vi "mod_Continuous BB-QAM generation.vi"(0 "Bit stream":T1(tab), 1 "Symbol Rate, Hz":dbl=1.0 format="%.2f", 2 "QAM system parameters":T2={"samples per symbol (16)"=16, "symbol map"=[]} {"symbol map" format="%.3f"}, 5 "PN Sequence Order":i32=9, 9 "user base bit pattern":i8[](array[numeric]), 11 "error in (no error)":errorcluster, 12 "filter parameters":T3={"Alpha"=0.5, "Filter Length"=6, "TX Filter"=enum."Root Raised Cos"} {"Alpha" format="%.2f"}, 13 "Path":path) -> (4 "output complex waveform":T4 {"Y" format="%.3f"; "dt" format="%^.2e"; "t0" format="%.4f"}, 6 "modulated bitstream":i8[](array[numeric]), 8 "pulse shaping filter coefficients":dbl[](array[numeric]) format="%.2f", 10 "matched filter coefficients":dbl[](array[numeric]) format="%.2f", 15 "error out":errorcluster)   [LabVIEW 2020, in "niDMT.lvlib"]
uses:
  <vilib>/addons/Modulation/niDMT.lvlib
  <vilib>/addons/Modulation/Analog/controls/Complex Data Waveform.ctl
  <vilib>/addons/Modulation/Digital/Support/Controls/QAM System Parameters.ctl
  <vilib>/addons/Modulation/Digital/General/MT Generate Bits (Galois, PN Order).vi
  <vilib>/addons/Modulation/Digital/Support/Common/Validators/mod_Generate Bits Validate.vi
  <vilib>/addons/Modulation/Analog/support/mod_Set Error Source.vi
  <vilib>/addons/Modulation/Digital/General/subVIs/mod_Generate Bits PN Sequence.vi
  <vilib>/addons/Modulation/Digital/General/MT Generate Bits (User Defined).vi
  <vilib>/Utility/file.llb/Read From Spreadsheet File (DBL).vi
  <vilib>/addons/Modulation/Digital/Support/Common/Validators/mod_Generate Filter Coefficients Validate.vi
  <vilib>/addons/Modulation/Digital/General/subVIs/mod_Generate Filter Coefficients.vi
  <vilib>/addons/Modulation/niAMT.lvlib
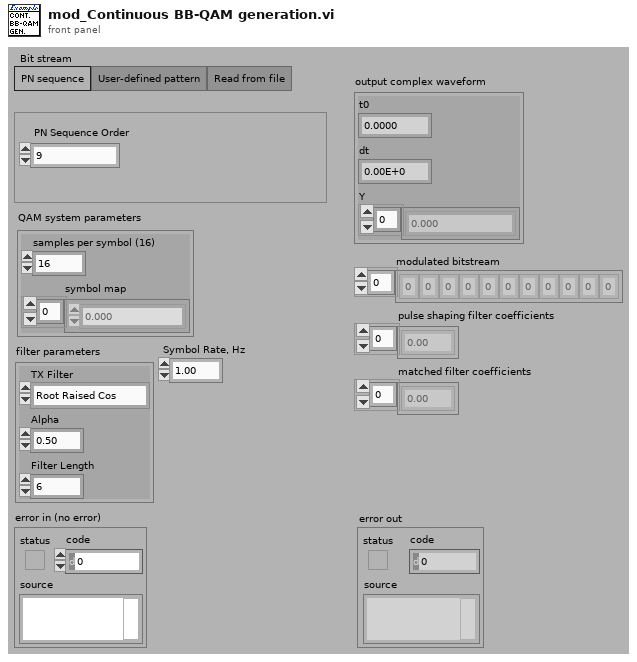
[diagram p1: front panel]
types:
  T1 = enum32{"PN sequence", "User-defined pattern", "Read from file"}
  T2 = typedef "niDMT.lvlib/QAM System Parameters.ctl" = cluster{"samples per symbol (16)":i32, "symbol map":cdb[]}
  T3 = cluster{"Alpha":dbl, "Filter Length":i32, "TX Filter":enum16{"none", "Raised Cosine", "Root Raised Cos", "Gaussian"}}
  T4 = typedef "niAMT.lvlib/Complex Data Waveform.ctl" = cluster{"t0":dbl, "dt":dbl, "Y":cdb[]}
  T5 = enum16{"none", "Raised Cosine", "Root Raised Cos", "Gaussian"}
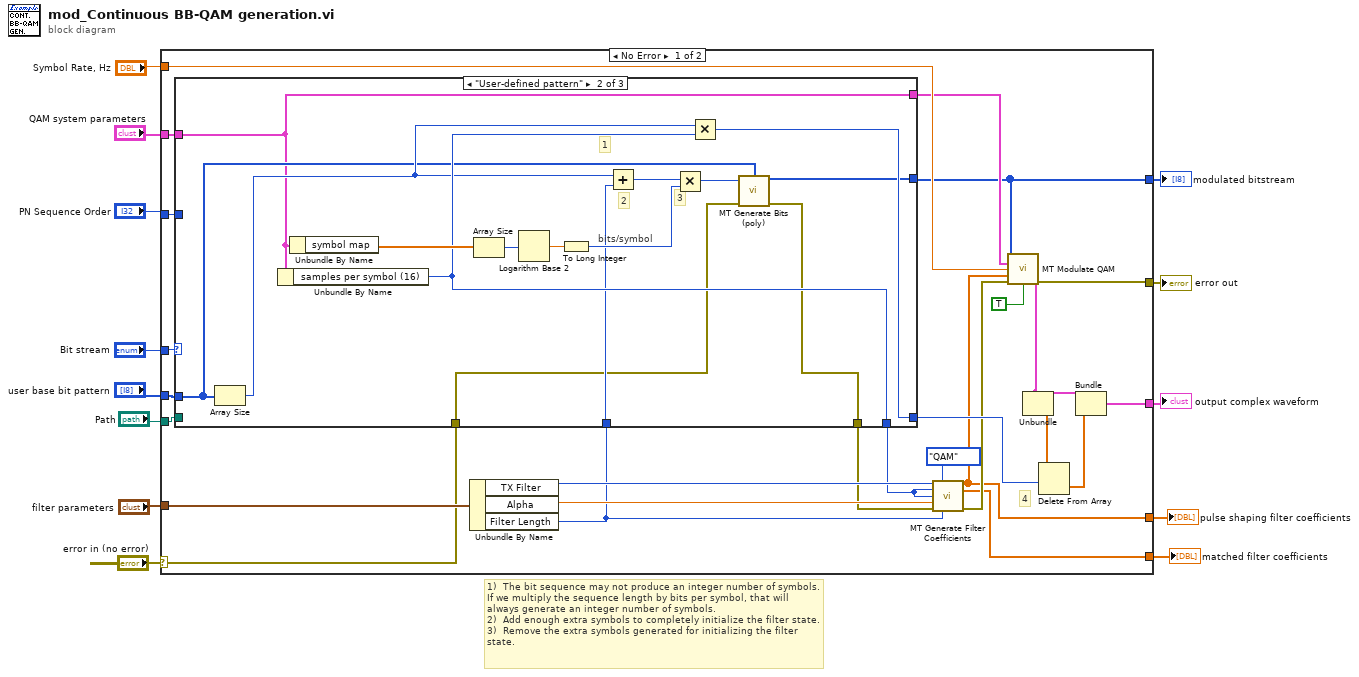
[diagram p0: block diagram]
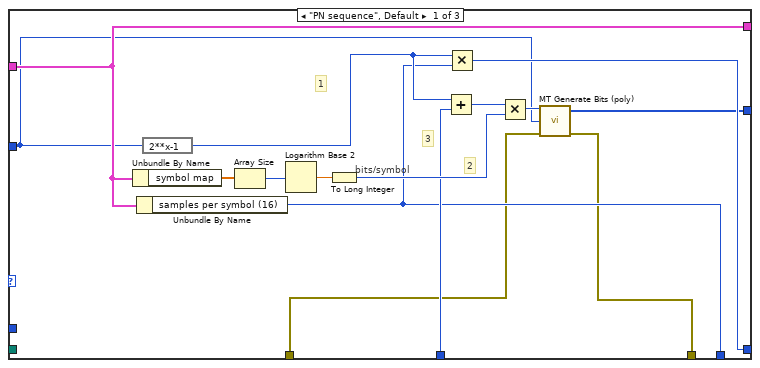
[diagram p2: hidden frame]
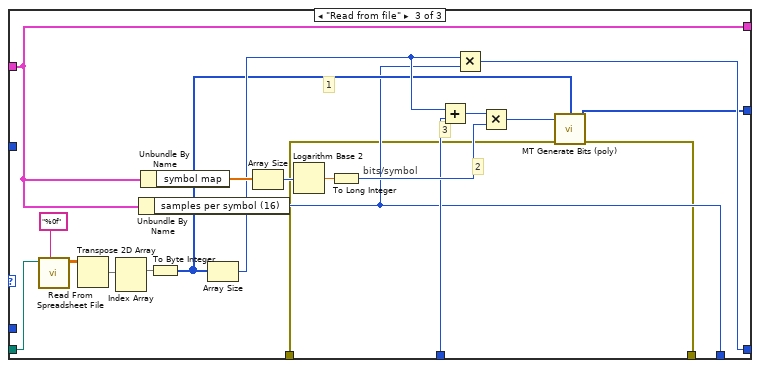
[diagram p3: hidden frame]
diagram:
  # "1)  The bit sequence may not produce an integer number of symbols.  If we multiply the sequence length by bits per symbol, that will always generate an integer number of symbols. \n2)  Add enough extra symbols to completely initialize the filter state.\n3)  Remove the extra symbols generated for initializing the filter state."
  n1 = case shown="No Error" "error in (no error)" {
    selector: "error in (no error)" -> [w19 w90]
    tunnel: [w39 _] -> w13
    tunnel: [w38 w90] -> w12
    tunnel: "Symbol Rate, Hz" -> [w35 _]
    tunnel: "PN Sequence Order" -> [w25 _]
    tunnel: "user base bit pattern" -> [w34 _]
    tunnel: "Bit stream" -> [w27 _]
    tunnel: "filter parameters" -> [w33 _]
    tunnel: "QAM system parameters" -> [w24 _]
    tunnel: "Path" -> [w26 _]
    tunnel: [w16 _] -> w3
    tunnel: [w15 _] -> w2
    tunnel: [w14 _] -> w1
    frame No Error {
      # "4"
      n2 = Unbundle By Name(w33) -> ("TX Filter"=w36:T5, "Alpha"=w37:dbl, "Filter Length"=w17:i32)
      n3 = case shown="\"User-defined pattern\"" w27 {
        tunnel: w34 -> [_ w59 _]
        tunnel: w25 -> [w42 _ _]
        tunnel: w26 -> [_ _ w86]
        tunnel: w24 -> [w45 w57 w73]
        tunnel: [w46 w63 w75] -> w23
        tunnel: [w44 w62 w74] -> w22
        tunnel: w17 -> [w47 w60 w76]
        tunnel: [w43 w58 w72] -> w16
        tunnel: [w45 w57 w73] -> w21
        tunnel: w19 -> [w41 w56 w71]
        tunnel: [w40 w55 w70] -> w18
        frame "PN sequence", Default {
          # "2"
          # "1"
          # "3"
          # "bits/symbol"
          n4 = Unbundle By Name(w45) -> ("symbol map"=w49:cdb[])
          n5 = Unbundle By Name(w45) -> ("samples per symbol (16)"=w46:i32)
          n6 = expression code="2**x-1"(w42) -> (w48:i32)
          n7 = Array Size(array=w49) -> (size(s)=w50:i32)
          n8 = Logarithm Base 2(1:w50) -> (0:w51:dbl)
          n9 = To Long Integer(number=w51) -> (32bit integer=w52:i32)
          n10 = Add(x=w48, y=w47) -> (x+y=w53:i32)
          n11 = Multiply(x=w48, y=w46) -> (x*y=w44:i32)
          n12 = Multiply(x=w53, y=w52) -> (x*y=w54:i32)
          n13 = call-poly <vilib>:"MT Generate Bits (poly).vi"("total bits (128)"=w54, "PN sequence order (9)"=w42, "error in (no error)"=w41) -> ("output bit stream"=w43:i8[], "error out"=w40:errorcluster)  [unwired: 2 in, 9 out]
        }
        frame "User-defined pattern" {
          # "2"
          # "1"
          # "3"
          # "bits/symbol"
          n14 = Array Size(array=w59) -> (size(s)=w61:i32)
          n15 = Unbundle By Name(w57) -> ("samples per symbol (16)"=w63:i32)
          n16 = Unbundle By Name(w57) -> ("symbol map"=w64:cdb[])
          n17 = Array Size(array=w64) -> (size(s)=w65:i32)
          n18 = Logarithm Base 2(1:w65) -> (0:w66:dbl)
          n19 = To Long Integer(number=w66) -> (32bit integer=w67:i32)
          n20 = Add(x=w61, y=w60) -> (x+y=w68:i32)
          n21 = Multiply(x=w68, y=w67) -> (x*y=w69:i32)
          n22 = Multiply(x=w61, y=w63) -> (x*y=w62:i32)
          n23 = call-poly <vilib>:"MT Generate Bits (poly).vi"("total bits (128)"=w69, "user base bit pattern"=w59, "error in (no error)"=w56) -> ("output bit stream"=w58:i8[], "error out"=w55:errorcluster)  [unwired: 2 in, 9 out]
        }
        frame "Read from file" {
          # "2"
          # "1"
          # "3"
          # "bits/symbol"
          n24 = call-poly <vilib>:"Read From Spreadsheet File.vi"("format (%.3f)"="%0f", "file path (dialog if empty)"=w86) -> ("all rows"=w87:dbl[][])  [unwired: 2 in, 7 out]
          n25 = Transpose 2D Array(2D array=w87) -> (transposed array=w88:dbl[][])
          n26 = Index Array(array=w88) -> (element=w89:dbl[])  [unwired: 2 in]
          n27 = Unbundle By Name(w73) -> ("samples per symbol (16)"=w75:i32)
          n28 = Unbundle By Name(w73) -> ("symbol map"=w79:cdb[])
          n29 = To Byte Integer(number=w89) -> (8bit integer=w77:i8[])
          n30 = Array Size(array=w77) -> (size(s)=w78:i32)
          n31 = Array Size(array=w79) -> (size(s)=w80:i32)
          n32 = Logarithm Base 2(1:w80) -> (0:w81:dbl)
          n33 = To Long Integer(number=w81) -> (32bit integer=w82:i32)
          n34 = Add(x=w78, y=w76) -> (x+y=w83:i32)
          n35 = Multiply(x=w78, y=w75) -> (x*y=w74:i32)
          n36 = Multiply(x=w83, y=w82) -> (x*y=w84:i32)
          n37 = call-poly <vilib>:"MT Generate Bits (poly).vi"("total bits (128)"=w84, "user base bit pattern"=w77, "error in (no error)"=w71) -> ("output bit stream"=w72:i8[], "error out"=w70:errorcluster)  [unwired: 2 in, 9 out]
        }
      }
      n38 = call <vilib>:"MT Generate Filter Coefficients.vi"("pulse shaping filter (none)"=w36, "modulation type"=enum16{"FSK", "PSK", "QAM", "MSK", "PAM", "ASK"}."QAM", "pulse shaping samples per symbol (16)"=w23, "matched samples per symbol (16)"=w23, "filter parameter"=w37, "error in (no error)"=w18, "filter length (symbols)"=w17) -> ("pulse shaping filter coefficients"=w15:dbl[], "matched filter coefficients"=w14:dbl[], "error out"=w20:errorcluster)  [unwired: 6 out]
      n39 = call <vilib>:"MT Modulate QAM.vi"("input bit stream"=w16, "QAM system parameters"=w21, "symbol rate (Hz)"=w35, "pulse shaping filter coefficients"=w15, "error in (no error)"=w20, "reset? (T)"=TRUE ("Reset (T)")) -> ("output complex waveform"=w32:T4, "error out"=w38:errorcluster)  [unwired: 1 in, 7 out]
      n40 = Unbundle(w32) -> ("Y"=w29:cdb[])  [unwired: 2 out]
      n41 = Delete From Array(array=w29, length=w22) -> (deleted portion=w30:cdb[])  [unwired: 1 in, 1 out]
      n42 = Bundle(cluster=w32, "Y"=w30) -> (w39:T4)  [unwired: 2 out]
    }
    frame Error {
    }
  }
  "error out" <- w12
  "output complex waveform" <- w13
  "modulated bitstream" <- w3
  "pulse shaping filter coefficients" <- w2
  "matched filter coefficients" <- w1
